vi "Start_just_treatment.vi"(1 "Graph refs":T2, 8 "error in (no error)":errorcluster, 9 "Slider cluster":T4, 10 "extra refs":T1, 11 "Control-Client in":refnum<class "Control-Client.lvclass">) -> (0 "error out":errorcluster, 3 "Control-Client out":refnum<class "Control-Client.lvclass">)   [LabVIEW 2020, in "Control-Client.lvclass"]
uses:
  Control-Client.lvclass
  C:/dev/TRANCON/Classes/GeneralFunctionality/GeneralFunctionality.lvclass
  dependecies/ControlsVIs/Clusters-def/Graphs_ref_Client.ctl
  dependecies/ControlsVIs/Clusters-def/graphs_TR.ctl
  dependecies/ControlsVIs/Clusters-def/Message types.ctl
  Control-Client.lvclass/Control-Client.ctl
  GeneralFunctionality/GeneralFunctionality.lvclass/GeneralFunctionality.ctl
  GeneralFunctionality/GeneralFunctionality.lvclass
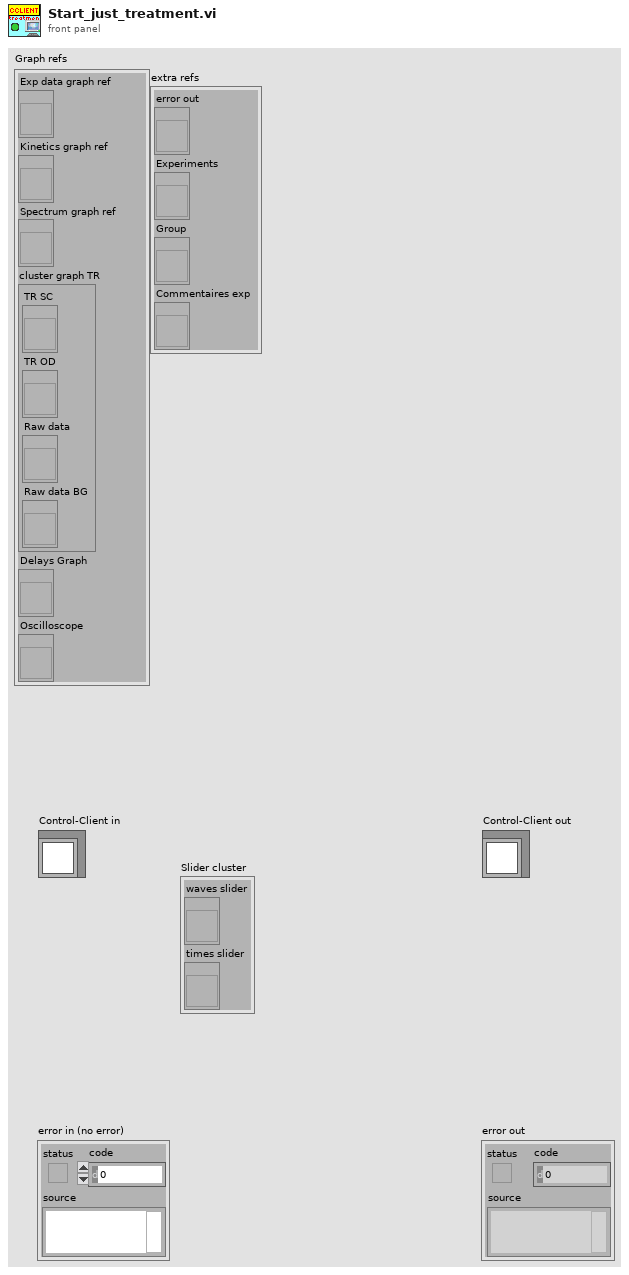
[diagram p1: front panel]
types:
  T1 = cluster{"error out":refnum<vi>, "Experiments":refnum<vi>, "Group":refnum<vi>, "Commentaires exp":refnum<vi>}
  T2 = typedef "Control-Client.lvclass/Graphs_ref_Client.ctl" = cluster{"Exp data graph ref":refnum<vi>, "Kinetics graph ref":refnum<vi>, "Spectrum graph ref":refnum<vi>, "cluster graph TR":T3, "Delays Graph":refnum<vi>, "Oscilloscope":refnum<vi>}
  T3 = typedef "graphs_TR.ctl" = cluster{"TR SC":refnum<vi>, "TR OD":refnum<vi>, "Raw data":refnum<vi>, "Raw data BG":refnum<vi>}
  T4 = cluster{"waves slider":refnum<vi>, "times slider":refnum<vi>}
  T5 = typedef "Message types.ctl" = string
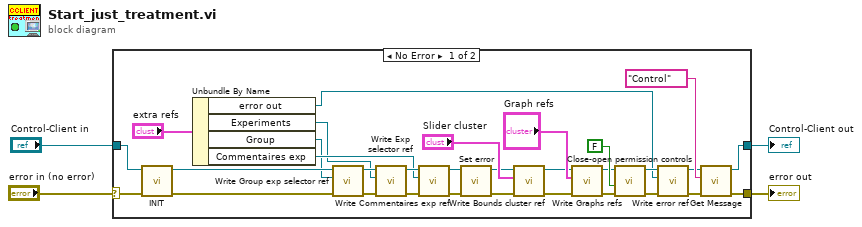
[diagram p0: block diagram]
diagram:
  n1 = case shown="No Error" "error in (no error)" {
    selector: "error in (no error)" -> [w35 w37]
    tunnel: [w5 w37] -> w3
    tunnel: [w6 w36] -> w1
    tunnel: "Control-Client in" -> [w26 w36]
    frame No Error {
      n2 = call-dynamic "INIT.vi"("error in (no error)"=w35, "Control-Client in"=w26) -> ("error out"=w34:errorcluster, "Control-Client out"=w33:refnum<class "Control-Client.lvclass">)  [unwired: 8 in]
      n3 = Unbundle By Name("extra refs") -> ("error out"=w17:refnum<vi>, "Experiments"=w14:refnum<vi>, "Group"=w15:refnum<vi>, "Commentaires exp"=w16:refnum<vi>)
      n4 = call "Write Group exp selector ref.vi"("error in (no error)"=w34, "Group exp selector ref"=w15, "Control-Client in"=w33) -> ("error out"=w31:errorcluster, "Control-Client out"=w32:refnum<class "Control-Client.lvclass">)  [unwired: 7 in]
      n5 = call "Write Exp selector ref.vi"("error in (no error)"=w31, "Exp selector ref"=w14, "Control-Client in"=w32) -> ("error out"=w30:errorcluster, "Control-Client out"=w29:refnum<class "Control-Client.lvclass">)  [unwired: 7 in]
      n6 = call "Write Commentaires exp ref.vi"("error in (no error)"=w30, "Commentaires exp"=w16, "Control-Client in"=w29) -> ("error out"=w27:errorcluster, "Control-Client out"=w28:refnum<class "Control-Client.lvclass">)  [unwired: 7 in]
      n7 = call "Set error.vi"("error in (no error)"=w27, "Control-Client in"=w28) -> ("error out"=w9:errorcluster, "Control-Client out"=w10:refnum<class "Control-Client.lvclass">)  [unwired: 8 in]
      n8 = call "Write Bounds cluster ref.vi"("error in (no error)"=w9, "Bounds cluster"="Slider cluster", "Control-Client in"=w10) -> ("error out"=w7:errorcluster, "Control-Client out"=w8:refnum<class "Control-Client.lvclass">)  [unwired: 7 in]
      n9 = call "Write Graphs refs.vi"("error in (no error)"=w7, "Graph refs"="Graph refs", "Control-Client in"=w8) -> ("error out"=w22:errorcluster, "Control-Client out"=w21:refnum<class "Control-Client.lvclass">)  [unwired: 7 in]
      n10 = call "Close-open permission controls.vi"("error in (no error)"=w22, "Boolean"=FALSE, "Control-Client in"=w21) -> ("error out"=w19:errorcluster, "Control-Client out"=w20:refnum<class "Control-Client.lvclass">)  [unwired: 7 in]
      n11 = call "Write error ref.vi"("error in (no error)"=w19, "error"=w17, "GeneralFunctionality in"=w20) -> ("error out"=w11:errorcluster, "GeneralFunctionality out"=w12:refnum<class "Control-Client.lvclass">)  [unwired: 7 in]
      n12 = call "Get Message.vi"("error in (no error)"=w11, "Message type"=T5 "Control", "GeneralFunctionality en entrée"=w12) -> ("error out"=w5:errorcluster, "GeneralFunctionality en sortie"=w6:refnum<class "Control-Client.lvclass">)  [unwired: 6 in, 1 out]
    }
    frame Error {
    }
  }
  "error out" <- w3
  "Control-Client out" <- w1
